vi "Utrasone_sensor.vi"() -> ()   [LabVIEW 2024]
uses:
  Control 3.ctl
  <vilib>/Instr/_visa.llb/VISA Configure Serial Port (Instr).vi
  <vilib>/Utility/file.llb/Write Delimited Spreadsheet (DBL).vi
panel:
  in  "file path (dialog if empty)":path
  out "state":string
  in  "Ingestelde Temperatuur":dbl
  out "motorPWM 2":string
  out "Waveform Chart":dbl(graph)
  out "remaining string":string
  out "inputArray":dbl[](array[numeric])
  in  "VISA resource name":refnum<visa-resource-name>
  in  "Stop":bool
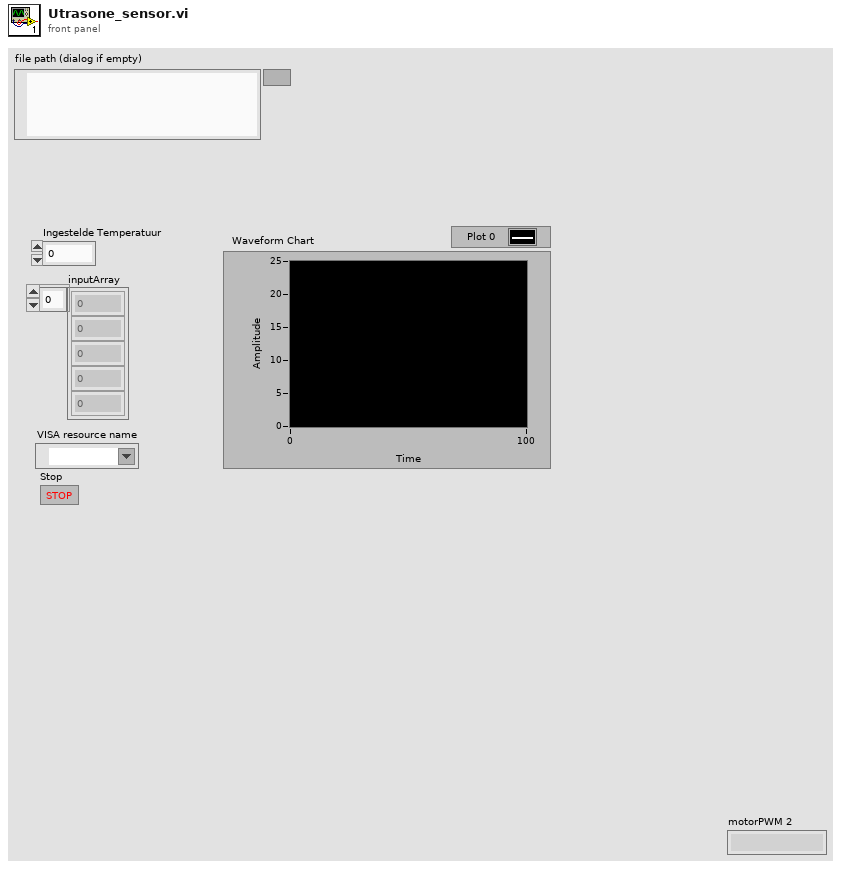
[diagram p1: front panel]
types:
  T1 = typedef "Control 3.ctl" = enum16{"humidity", "Temperatuur", "hic", "potVal", "btnVal"}
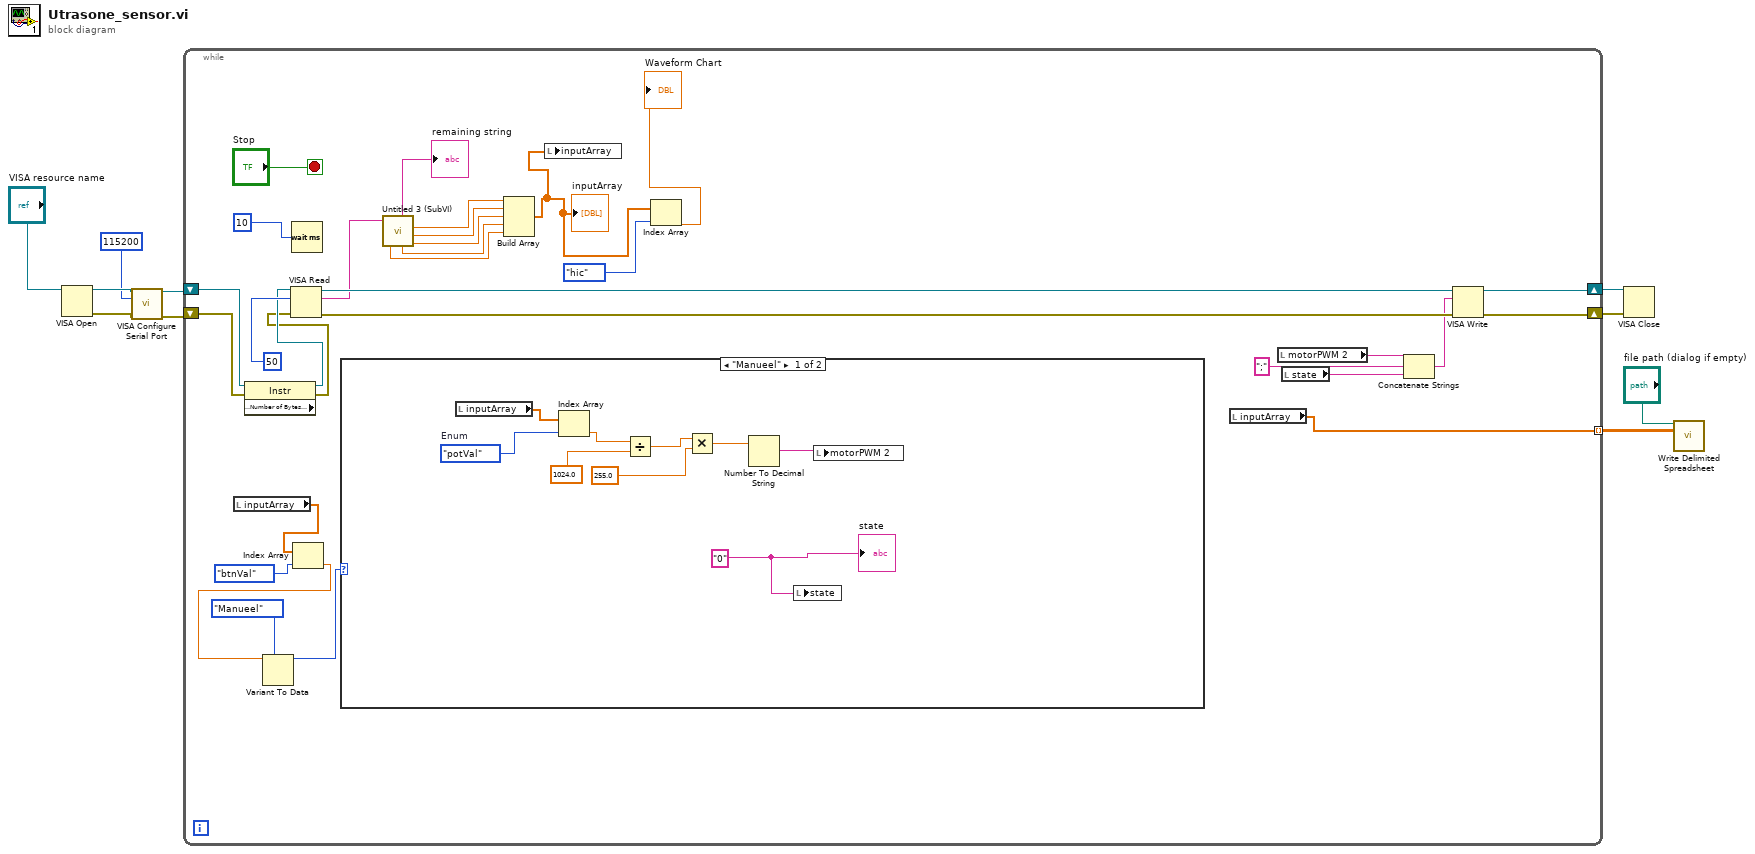
[diagram p0: block diagram]
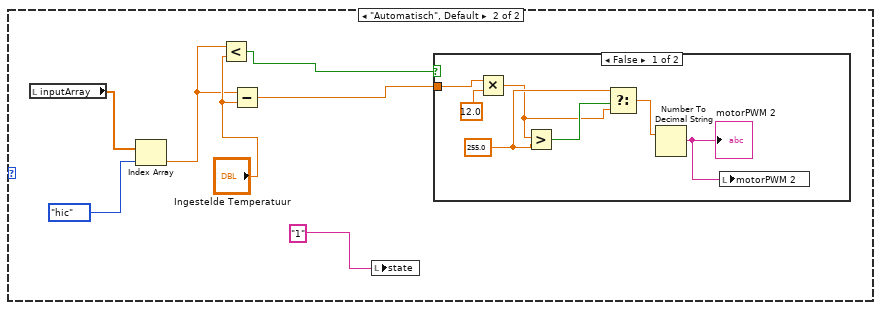
[diagram p2: hidden frame]
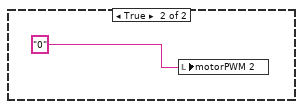
[diagram p3: hidden frame]
diagram:
  n1 = VISA Open(VISA resource name="VISA resource name") -> (VISA resource name=w7:refnum<visa-resource-name>, error out=w5:errorcluster)  [unwired: 4 in]
  n2 = call-poly "VISA Configure Serial Port"("VISA resource name"=w7, "baud rate (9600)"=u32 115200, "error in (no error)"=w5) -> ("VISA resource name out"=w6:refnum<visa-resource-name>, "error out"=w4:errorcluster)  [unwired: 11 in]
  n3 = while {
    shift-right: [w36] -> w10
    shift-left: w6 -> [w34]
    shift-right: [w35] -> w9
    shift-left: w4 -> [w33]
    tunnel: [w11] -> w2 mode=indexing
    stop <- "Stop" stop-if-true
    n4 = local read "inputArray"() -> (w23:dbl[])
    n5 = property class="Instr" props=["Serial Settings:Number of Bytes at Serial Port"](reference=w34, error in=w33) -> (reference out=w32:refnum<visa-resource-name>, error out=w31:errorcluster)  [unwired: 1 out]
    n6 = VISA Read(VISA resource name=w32, byte count=u32 50, error in (no error)=w31) -> (VISA resource name out=w38:refnum<visa-resource-name>, read buffer=w29:string, error out=w37:errorcluster)  [unwired: 1 out]
    n7 = Wait (ms)(milliseconds to wait=u32 10) -> ()  [unwired: 1 out]
    n8 = Index Array(array=w23, index=Control_3."btnVal") -> (element=w13:dbl)
    n9 = Variant To Data(type=enum16{"Manueel", "Automatisch"}."Manueel", Variant=w13) -> (data=w12:enum16{"Manueel", "Automatisch"})  [unwired: 1 in, 1 out]
    n10 = case shown="\"Manueel\"" w12 {
      frame "Manueel" {
        w42 = "0" ("String")
        w49 = Control_3."potVal"  # Enum
        n11 = local read "inputArray"() -> (w50:dbl[])
        n12 = Index Array(array=w50, index=w49) -> (element=w48:dbl)
        n13 = Divide(x=w48, y=1024.0) -> (x/y=w46:dbl)
        n14 = Multiply(x=w46, y=255.0) -> (x*y=w44:dbl)
        n15 = Number To Decimal String(number=w44) -> (decimal integer string=w43:string)  [unwired: 1 in]
        n16 = local write "state"(w42) -> ()
        n17 = local write "motorPWM 2"(w43) -> ()
        "state" <- w42
      }
      frame "Automatisch", Default {
        n18 = local read "inputArray"() -> (w53:dbl[])
        n19 = Index Array(array=w53, index=Control_3."hic" ("Enum")) -> (element=w52:dbl)
        n20 = Less?(x=w52, y="Ingestelde Temperatuur") -> (x < y?=w55:bool)
        n21 = Subtract(x=w52, y="Ingestelde Temperatuur") -> (x-y=w57:dbl)
        n22 = local write "state"("1" ("String")) -> ()
        n23 = case shown="False" w55 {
          tunnel: w57 -> [w64 _]
          frame False {
            w61 = 255.0 ("y")
            n24 = Multiply(x=w64, y=12.0) -> (x*y=w60:dbl)
            n25 = Greater?(x=w60, y=w61) -> (0:w62:bool)
            n26 = Select(t=w61, s=w62, f=w60) -> (s? t:f=w59:dbl)
            n27 = Number To Decimal String(number=w59) -> (decimal integer string=w58:string)  [unwired: 1 in]
            "motorPWM 2" <- w58
            n28 = local write "motorPWM 2"(w58) -> ()
          }
          frame True {
            n29 = local write "motorPWM 2"("0" ("String")) -> ()
          }
        }
      }
    }
    n30 = call "Untitled 3 (SubVI).vi"("input string"=w29) -> ("btnVal"=w17:dbl, "remaining string"=→"remaining string":string, "potVal"=w18:dbl, "Humdity"=w21:dbl, "Temperatuur"=w20:dbl, "Hic"=w19:dbl)  [unwired: 1 in]
    n31 = Build Array(w21, w20, w19, w18, w17) -> (w16:dbl[])
    "inputArray" <- w16
    n32 = local write "inputArray"(w16) -> ()
    n33 = Index Array(array=w16, index=Control_3."hic" ("Enum")) -> (element=→"Waveform Chart":dbl)
    n34 = local read "inputArray"() -> (w11:dbl[])
    n35 = local read "motorPWM 2"() -> (w25:string)
    n36 = local read "state"() -> (w15:string)
    n37 = Concatenate Strings(w25, ";" ("string"), w15) -> (w26:string)
    n38 = VISA Write(VISA resource name=w38, write buffer=w26, error in (no error)=w37) -> (VISA resource name out=w36:refnum<visa-resource-name>, error out=w35:errorcluster)  [unwired: 1 out]
  }
  n39 = VISA Close(VISA resource name=w10, error in (no error)=w9) -> ()  [unwired: 1 out]
  n40 = call-poly <vilib>:"Write Delimited Spreadsheet.vi"("file path (dialog if empty)"="file path (dialog if empty)", "2D data"=w2) -> ()  [unwired: 12 in, 2 out]
